vi "Express_Filter.vi"() -> ()   [LabVIEW 2010]
doc: "Example of Generate and Display template.\n\nThis VI generates a sine wave with a frequency of 10 Hz and an amplitude of 10 volts with white noise of 3 volts of amplitude. You can customize these parameters using the controls Simulated frequency, Simulated amplitude and Simulated noise amplitude.\n\nThe signal then goes through a 5 order elliptic low pass IIR filter in order to filter the noise. The cut off frequency of the filter is 15 Hz. Both the original and the filtered signal are displayed.\n\nPush the stop button to halt the execution."
panel:
  in  "Simulated amplitude":dbl=10.0 min=0.0 format="%0.2f"
  in  "Simulated noise amplitude":dbl=3.0 min=0.0 format="%0.2f"
  in  "Simulated frequency":dbl=10.0 min=0.0 format="%0.2f"
  out "Filtered  Amplitude":dbl
  out "Filtered Frequency":dbl
  out "Frequency":dbl
  out "Amplitude":dbl
  out "Filtered Signal":dynamicdata(graph)
  out "Simulated Signal":dynamicdata(graph)
  in  "stop":bool
  # "Go to File»VI Properties»Documentation for a detailed explanation of this VI"
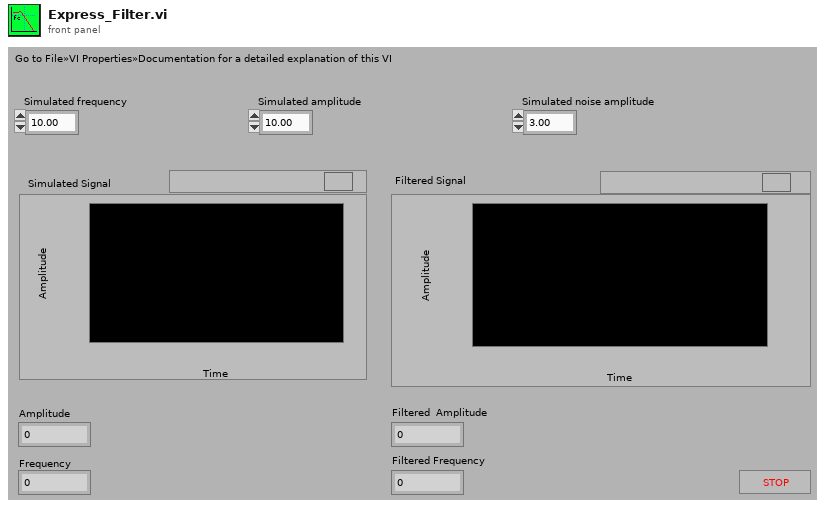
[diagram p1: front panel]
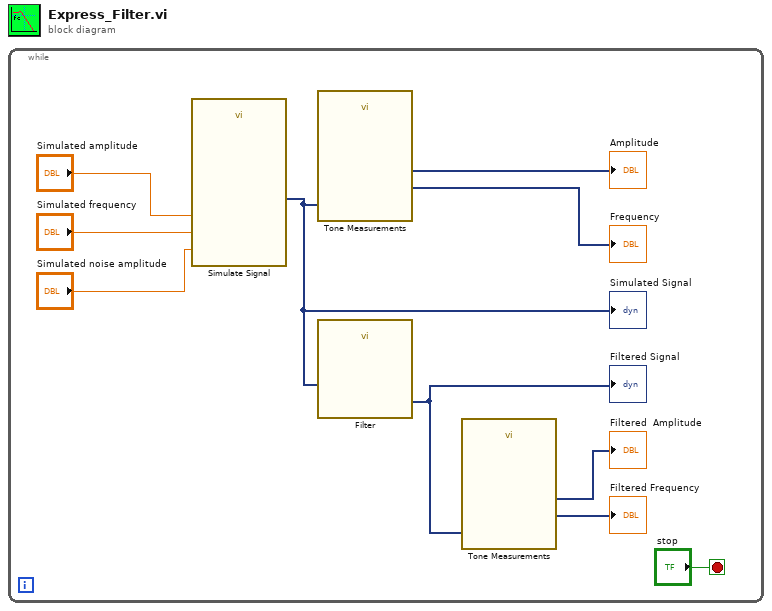
[diagram p0: block diagram]
diagram:
  n1 = while {
    stop <- "stop" stop-if-true
    n2 = call "Simulate Signal"("Frequency"="Simulated frequency", "Amplitude"="Simulated amplitude", "Noise amplitude"="Simulated noise amplitude") -> ("Sine with Uniform Noise"=w4:dynamicdata)  [unwired: 11 in, 1 out]
    "Simulated Signal" <- w4
    n3 = call "Tone Measurements"("Signals"=w4) -> ("Frequency"=→"Frequency":dynamicdata, "Amplitude"=→"Amplitude":dynamicdata)  [unwired: 7 in, 2 out]
    n4 = call "Filter"("Signal"=w4) -> ("Filtered Signal"=w7:dynamicdata)  [unwired: 9 in, 1 out]
    "Filtered Signal" <- w7
    n5 = call "Tone Measurements"("Signals"=w7) -> ("Frequency"=→"Filtered Frequency":dynamicdata, "Amplitude"=→"Filtered  Amplitude":dynamicdata)  [unwired: 7 in, 2 out]
  }
